vi "smgr2table.vi"(4 "t0":timestamp, 5 "Array 2":waveform(i16)[][](array[waveform]), 6 "detected phase (deg)":dbl, 7 "write2file":bool) -> (0 "error out":errorcluster, 1 "values":string[][](array[string]), 2 "captions":string[](array[string])=["фаза, градусы", "относит. время, мкс", "макс. A, мВ", "макс. B, мВ", "макс. C, мВ"], 3 "zipped path":path)   [LabVIEW 2010]
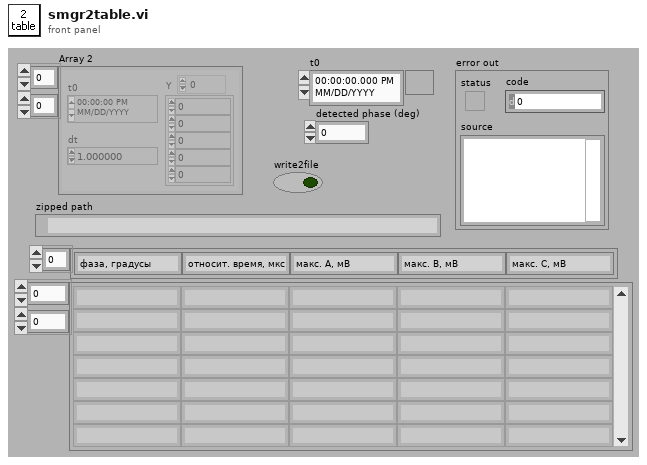
[diagram p1: front panel]
types:
  T1 = enum16{"open", "replace", "create", "open or create", "replace or create", "replace or create with confirmation"}
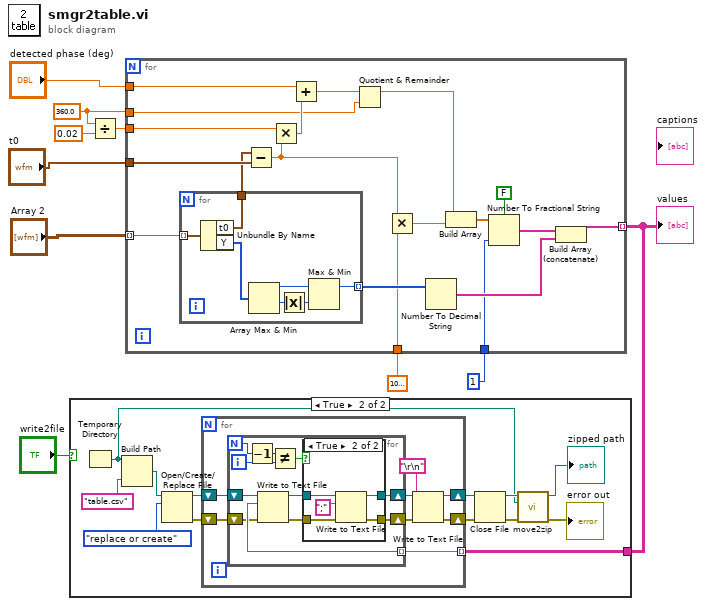
[diagram p0: block diagram]
diagram:
  w5 = 360.0 ("y")
  n1 = Divide(x=w5, y=0.02) -> (x/y=w4:dbl)
  n2 = for {
    tunnel: "Array 2" -> [w29] mode=indexing
    tunnel: [w27] -> w2 mode=indexing
    tunnel: "t0" -> [w24]
    tunnel: "detected phase (deg)" -> [w20]
    tunnel: w4 -> [w23]
    tunnel: 1000000.0 ("y") -> [w15]
    tunnel: i16 1 ("precision (6)") -> [w14]
    tunnel: w5 -> [w13]
    n3 = for {
      tunnel: w29 -> [w36] mode=indexing
      tunnel: [w32] -> w28 mode=indexing
      tunnel: [w31] -> w22
      n4 = Unbundle By Name(w36) -> ("t0"=w31:timestamp, "Y"=w30:i16[])
      n5 = Array Max & Min(array=w30) -> (max value=w35:i16, min value=w34:i16)  [unwired: 2 out]
      n6 = Absolute Value(x=w34) -> (abs(x)=w33:i16)
      n7 = Max & Min(x=w35, y=w33) -> (max(x,y)=w32:i16)  [unwired: 1 out]
    }
    n8 = Subtract(x=w22, y=w24) -> (x-y=w12:dbl)
    n9 = Multiply(x=w23, y=w12) -> (x*y=w21:dbl)
    n10 = Add(x=w20, y=w21) -> (x+y=w17:dbl)
    n11 = Quotient & Remainder(x=w17, y=w13) -> (x-y*floor(x/y)=w16:dbl)  [unwired: 1 out]
    n12 = Multiply(x=w12, y=w15) -> (x*y=w19:dbl)
    n13 = Number To Decimal String(number=w28) -> (decimal integer string=w26:string[])  [unwired: 1 in]
    n14 = Build Array(w16, w19) -> (w18:dbl[])
    n15 = Number To Fractional String(use system decimal point (T)=FALSE, number=w18, precision (6)=w14) -> (F-format string=w25:string[])  [unwired: 1 in]
    n16 = Build Array (concatenate)(w25, w26) -> (w27:string[])
  }
  "values" <- w2
  n17 = case shown="True" "write2file" {
    tunnel: w2 -> [_ w49]
    frame False {
    }
    frame True {
      n18 = Temporary Directory() -> (w39:path)
      n19 = Build Path(base path=w39, name or relative path="table.csv") -> (appended path=w41:path)
      n20 = Open/Create/Replace File(file path (use dialog)=w41, operation (0:open)=T1."replace or create") -> (refnum out=w43:refnum<file>, error out=w44:errorcluster)  [unwired: 4 in, 1 out]
      n21 = for {
        tunnel: w49 -> [w57] mode=indexing
        shift-right: [w51] -> w47
        shift-left: w44 -> [w50]
        shift-right: [w53] -> w46
        shift-left: w43 -> [w52]
        n22 = for {
          N -> [w67]
          tunnel: w57 -> [w62] mode=indexing
          shift-right: [w60] -> w56
          shift-left: w50 -> [w59]
          shift-right: [w58] -> w55
          shift-left: w52 -> [w68]
          i -> [w66]
          n23 = Decrement(x=w67) -> (x-1=w65:i32)
          n24 = Write to Text File(file (use dialog)=w68, text=w62, error in=w59) -> (refnum out=w61:refnum<file>, error out=w64:errorcluster)  [unwired: 1 in, 1 out]
          n25 = Not Equal?(x=w65, y=w66) -> (x != y?=w63:bool)
          n26 = case shown="True" w63 {
            tunnel: w64 -> [w70 w75]
            tunnel: w61 -> [w69 w73]
            tunnel: [w70 w72] -> w60
            tunnel: [w69 w71] -> w58
            frame False {
            }
            frame True {
              n27 = Write to Text File(file (use dialog)=w73, text=";", error in=w75) -> (refnum out=w71:refnum<file>, error out=w72:errorcluster)  [unwired: 1 in, 1 out]
            }
          }
        }
        n28 = Write to Text File(file (use dialog)=w55, text="\r\n", error in=w56) -> (refnum out=w53:refnum<file>, error out=w51:errorcluster)  [unwired: 1 in, 1 out]
      }
      n29 = Close File(refnum=w46, error in=w47) -> (path=w48:path, error out=w45:errorcluster)
      n30 = call "move2zip.vi"("error in"=w45, "dest dir"=w39, "source path"=w48) -> ("error out"=→"error out":errorcluster, "zipped path"=→"zipped path":path)  [unwired: 3 in]
    }
  }
